vi "Player Info.vi"(11 "Coward in":refnum<class "Coward.lvclass">) -> (0 "Defeat Speech":string, 1 "Victory Speech":string, 2 "Name":string, 3 "Coward out":refnum<class "Coward.lvclass">)   [LabVIEW 2015, in "Coward.lvclass"]
uses:
  Coward.lvclass
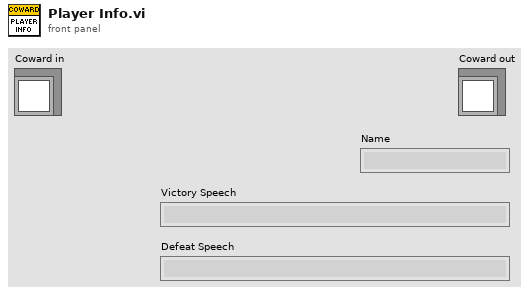
[diagram p1: front panel]
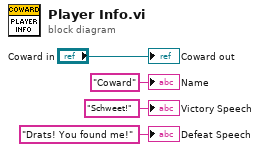
[diagram p0: block diagram]
diagram:
  "Coward out" <- "Coward in"
  "Name" <- "Coward" ("Name")
  "Victory Speech" <- "Schweet!" ("Victory Speech")
  "Defeat Speech" <- "Drats! You found me!" ("Defeat Speech")
